vi "Test General Error Propagation.vi"(11 "Test Case In":refnum<class "Test Open Xml.lvclass">) -> (0 "error out":errorcluster, 3 "Test Case Out":refnum<class "Test Open Xml.lvclass">)   [LabVIEW 2020, in "Test Open Xml.lvclass"]
uses:
  Test Open Xml.lvclass
  C:/Program Files/National Instruments/LabVIEW 2025/vi.lib/Astemes/LUnit/Test Case.lvclass
  <vilib>/Astemes/LUnit/Test Case.lvclass/Test Case.ctl
  Test Open Xml.lvclass/Test Open Xml.ctl
  <vilib>/Astemes/LUnit/Test Case.lvclass
  C:/Program Files/National Instruments/LabVIEW 2025/vi.lib/Astemes/LUnit/LUnit Runnable.lvclass
  D:/git/Open-Xml-LabVIEW/Test Open Xml/Test Open Xml.lvclass
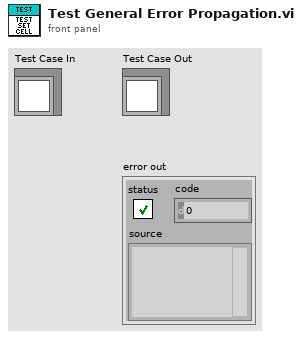
[diagram p1: front panel]
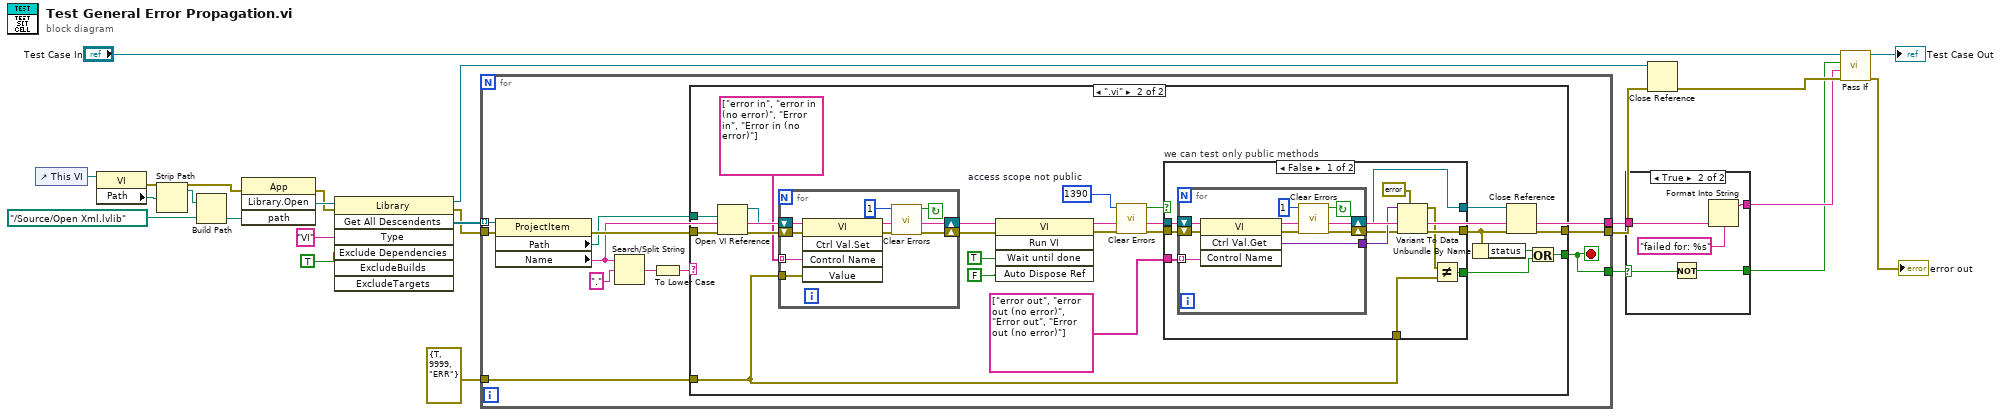
[diagram p0: block diagram]
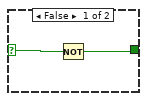
[diagram p4: hidden frame]
diagram:
  n1 = control-ref of="This VI"() -> (w6:refnum<vi>)
  n2 = property class="VI"(reference=w6) -> (error out=w3:errorcluster, "Path"=w4:path)  [unwired: 1 in, 1 out]
  n3 = Strip Path(path=w4) -> (stripped path=w2:path)  [unwired: 1 out]
  n4 = Build Path(base path=w2, name or relative path=path "../Source/Open Xml.lvlib" ("Path")) -> (appended path=w5:path)
  n5 = invoke class="App" method="Library.Open"(error in=w3, "path"=w5) -> (error out=w14:errorcluster, "Open Library"=w19:refnum<vi>)  [unwired: 2 in, 2 out]
  n6 = invoke class="Library" method="Get All Descendents"(reference=w19, error in=w14, "Type"="VI", "Exclude Dependencies"=TRUE ("ExcludeDependencies")) -> (reference out=w15:refnum<vi>, error out=w13:errorcluster, "All Descendents"=w16:refnum<vi>[])  [unwired: 3 in, 4 out]
  n7 = for {
    tunnel: w16 -> [w34] mode=indexing
    tunnel: w13 -> [w33]
    tunnel: [w29] -> w1
    tunnel: errorcluster {"status"=TRUE, "code"=9999, "source"="ERR"} ("error constant") -> [w31]
    tunnel: [w24] -> w10
    tunnel: [w30] -> w8
    stop <- w30 stop-if-true
    n8 = property class="ProjectItem"(reference=w34, error in=w33) -> (error out=w32:errorcluster, "Path"=w25:path, "Name"=w24:string)  [unwired: 1 out]
    n9 = Search/Split String(string=w24, search string/char (-)=".") -> (match + rest of string=w27:string)  [unwired: 1 in, 2 out]
    n10 = To Lower Case(string=w27) -> (all lower case string=w26:string)
    n11 = case shown="\".vi\"" w26 {
      tunnel: w32 -> [w35 w57]
      tunnel: w31 -> [_ w44]
      tunnel: [_ w54] -> w30
      tunnel: [w35 w37] -> w29
      tunnel: w25 -> [_ w43]
      frame Default {
      }
      frame ".vi" {
        w39 = 1390  # access scope not public
        n12 = Open VI Reference(vi path=w43, error in (no error)=w57) -> (vi reference=w50:refnum<vi>, error out=w51:errorcluster)  [unwired: 4 in]
        n13 = for {
          tunnel: string[] ["error in", "error in (no error)", "Error in", "Error in (no error)"] -> [w66] mode=indexing
          tunnel: w44 -> [w61]
          shift-right: [w60] -> w49
          shift-left: w51 -> [w65]
          shift-right: [w62] -> w48
          shift-left: w50 -> [w64]
          stop <- w58 continue-if-true
          n14 = invoke class="VI" method="Ctrl Val.Set"(reference=w64, error in=w65, "Control Name"=w66, "Value"=w61) -> (reference out=w62:refnum<vi>, error out=w63:errorcluster)  [unwired: 1 in, 3 out]
          n15 = call <vilib>:"Clear Errors.vi"("error in (no error)"=w63, "specific error code to clear (0: all)"=1) -> ("error out"=w60:errorcluster, "specific error cleared?"=w58:bool)  [unwired: 4 in]
        }
        n16 = invoke class="VI" method="Run VI"(reference=w48, error in=w49, "Wait until done"=TRUE ("Wait Until Done"), "Auto Dispose Ref"=FALSE ("Auto Dispose Reference")) -> (reference out=w46:refnum<vi>, error out=w47:errorcluster)  [unwired: 1 in, 3 out]
        n17 = call <vilib>:"Clear Errors.vi"("error in (no error)"=w47, "specific error code to clear (0: all)"=w39) -> ("error out"=w40:errorcluster, "specific error cleared?"=w38:bool)  [unwired: 4 in]
        n18 = case "we can test only public methods" shown="False" w38 {
          tunnel: [w77 _] -> w55
          tunnel: w46 -> [w76 w87]
          tunnel: [w75 w88] -> w45
          tunnel: w44 -> [w71 _]
          tunnel: string[] ["error out", "error out (no error)", "Error out", "Error out (no error)"] -> [w70 _]
          tunnel: w40 -> [w69 w88]
          tunnel: [w67 w87] -> w36
          frame False {
            n19 = for {
              tunnel: w70 -> [w83] mode=indexing
              tunnel: [w82] -> w74
              shift-right: [w80] -> w68
              shift-left: w69 -> [w86]
              shift-right: [w81] -> w67
              shift-left: w76 -> [w84]
              stop <- w78 continue-if-true
              n20 = invoke class="VI" method="Ctrl Val.Get"(reference=w84, error in=w86, "Control Name"=w83) -> (reference out=w81:refnum<vi>, error out=w85:errorcluster, "Get Control Value Variant"=w82:variant)  [unwired: 1 in, 1 out]
              n21 = call <vilib>:"Clear Errors.vi"("error in (no error)"=w85, "specific error code to clear (0: all)"=1) -> ("error out"=w80:errorcluster, "specific error cleared?"=w78:bool)  [unwired: 4 in]
            }
            n22 = Variant To Data(error in=w68, type=errorcluster {"status"=FALSE, "code"=0, "source"=""} ("error constant"), Variant=w74) -> (data=w73:errorcluster, error out=w75:errorcluster)
            n23 = Not Equal?(x=w73, y=w71) -> (x != y?=w77:bool)
          }
          frame True {
          }
        }
        n24 = Unbundle By Name(w45) -> ("status"=w56:bool)
        n25 = Close Reference(reference=w36, error in (no error)=w45) -> (error out=w37:errorcluster)
        n26 = Or(x=w56, y=w55) -> (x .or. y?=w54:bool)
      }
    }
  }
  n27 = case shown="True" w8 {
    selector: w8 -> [w90 w92]
    tunnel: w10 -> [_ w95]
    tunnel: [_ w93] -> w9
    tunnel: [w89 w91] -> w7
    frame False {
      n28 = Not(x=w90) -> (.not. x?=w89:bool)
    }
    frame True {
      n29 = Not(x=w92) -> (.not. x?=w91:bool)
      n30 = Format Into String(format string="failed for: %s", w95) -> (resulting string=w93:string)  [unwired: 2 in, 1 out]
    }
  }
  n31 = Close Reference(reference=w15, error in (no error)=w1) -> (error out=w11:errorcluster)
  n32 = call <vilib>:"Pass If.vi"("error in (no error)"=w11, "Message"=w9, "Pass?"=w7, "LUnit Test Case In"="Test Case In") -> ("error out"=→"error out":errorcluster, "LUnit Test Case Out"=→"Test Case Out":refnum<class "Test Open Xml.lvclass">)  [unwired: 6 in]
